vi "Problem1.4-SubVI.vi"(11 "Boolean\nInput":bool) -> (1 "Boolean":bool, 2 "Boolean 3":bool, 3 "Boolean 2":bool)   [LabVIEW 2018]
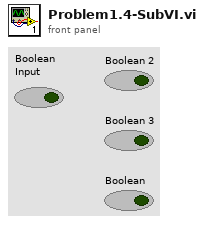
[diagram p1: front panel]
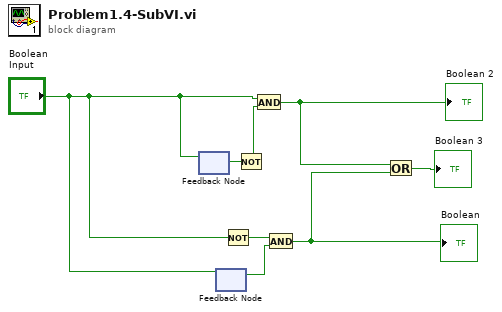
[diagram p0: block diagram]
diagram:
  n1 = feedback #1() -> (w1:bool)  [unwired: 1 in]
  n2 = feedback-in #1("Boolean\nInput") -> ()
  n3 = feedback #2() -> (w4:bool)  [unwired: 1 in]
  n4 = feedback-in #2("Boolean\nInput") -> ()
  n5 = Not(x="Boolean\nInput") -> (.not. x?=w3:bool)
  n6 = Not(x=w1) -> (.not. x?=w2:bool)
  n7 = And(x="Boolean\nInput", y=w2) -> (x .and. y?=w7:bool)
  "Boolean 2" <- w7
  n8 = And(x=w3, y=w4) -> (x .and. y?=w8:bool)
  "Boolean" <- w8
  n9 = Or(x=w7, y=w8) -> (x .or. y?=→"Boolean 3":bool)
